vi "VisualizeAppBase.vi"() -> ()   [LabVIEW 2017, in "Visualization.lvlib" / "VisualizeAppBase_class.lvclass"]
uses:
  VisualizeAppBase_class.lvclass
  Modules/AppModule/PublicAPI/Arguments/Broadcasts/clStatUpdate.ctl
  VisializeBase_class/Requests/clUserEventType.ctl
  <vilib>/event_ctls.llb/usereventprio.ctl
  <vilib>/Utility/error.llb/Error Cluster From Error Code.vi
  <vilib>/ErrorRing/Error Ring.xnode
  <userlib>/NIST/NISTErrorLib/NISTErrorLib.lvlib
  VisializeBase_class/VisualizeBase_class.lvclass
  Modules/AppModule/AppModule.lvlib
panel:
  out "Status Broadcasts":string
  out "Error Array":errorcluster[][](array[cluster])
  in  "QueName":string="VisAppQue"
  in  "btnStop":bool
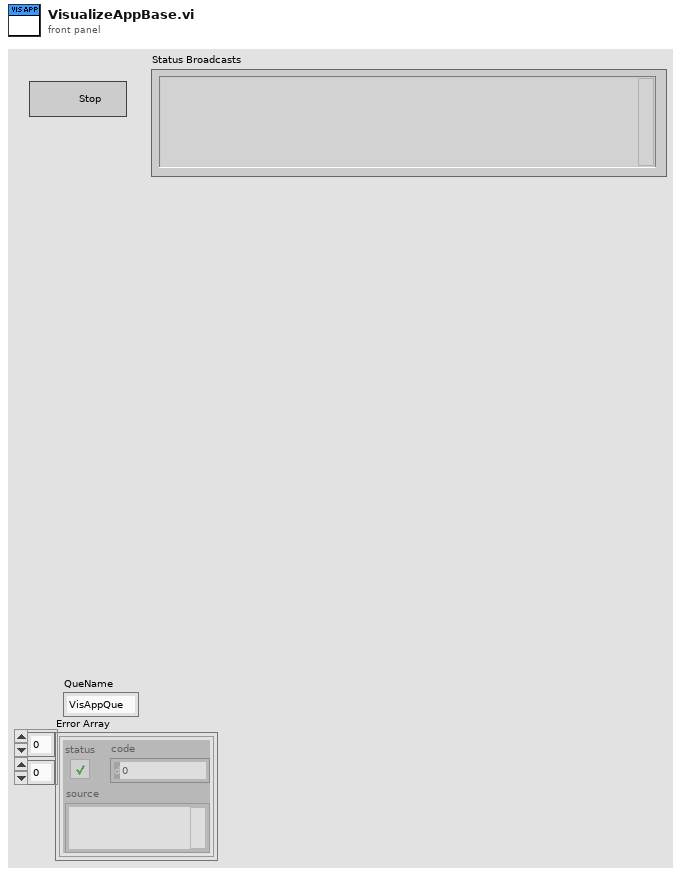
[diagram p1: front panel]
types:
  T1 = typedef "Visualization.lvlib/VisualizeBase_class.lvclass/clRequestEvents.ctl" = cluster{"StopRequest":refnum<user-event>}
  T2 = typedef "AppModule.lvlib/clBroadcastEvents.ctl" = cluster{"DidInit":refnum<user-event>, "StatusUpdate":refnum<user-event>, "ErrorReport":refnum<user-event>, "DidStop":refnum<user-event>, "PathToINI":refnum<user-event>, "InputData":refnum<user-event>, "OutputData":refnum<user-event>, "BcAppInfo":refnum<user-event>, "ConfigData":refnum<user-event>}
  T3 = typedef "Visualization.lvlib/VisualizeBase_class.lvclass/clUserEventType.ctl" = cluster{"BusIndex":i8, "Data":variant}
  T4 = typedef "usereventprio.ctl" = enum32{"high priority", "normal priority"}
  T5 = typedef "AppModule.lvlib/clStatUpdate.ctl" = cluster{"Status":string}
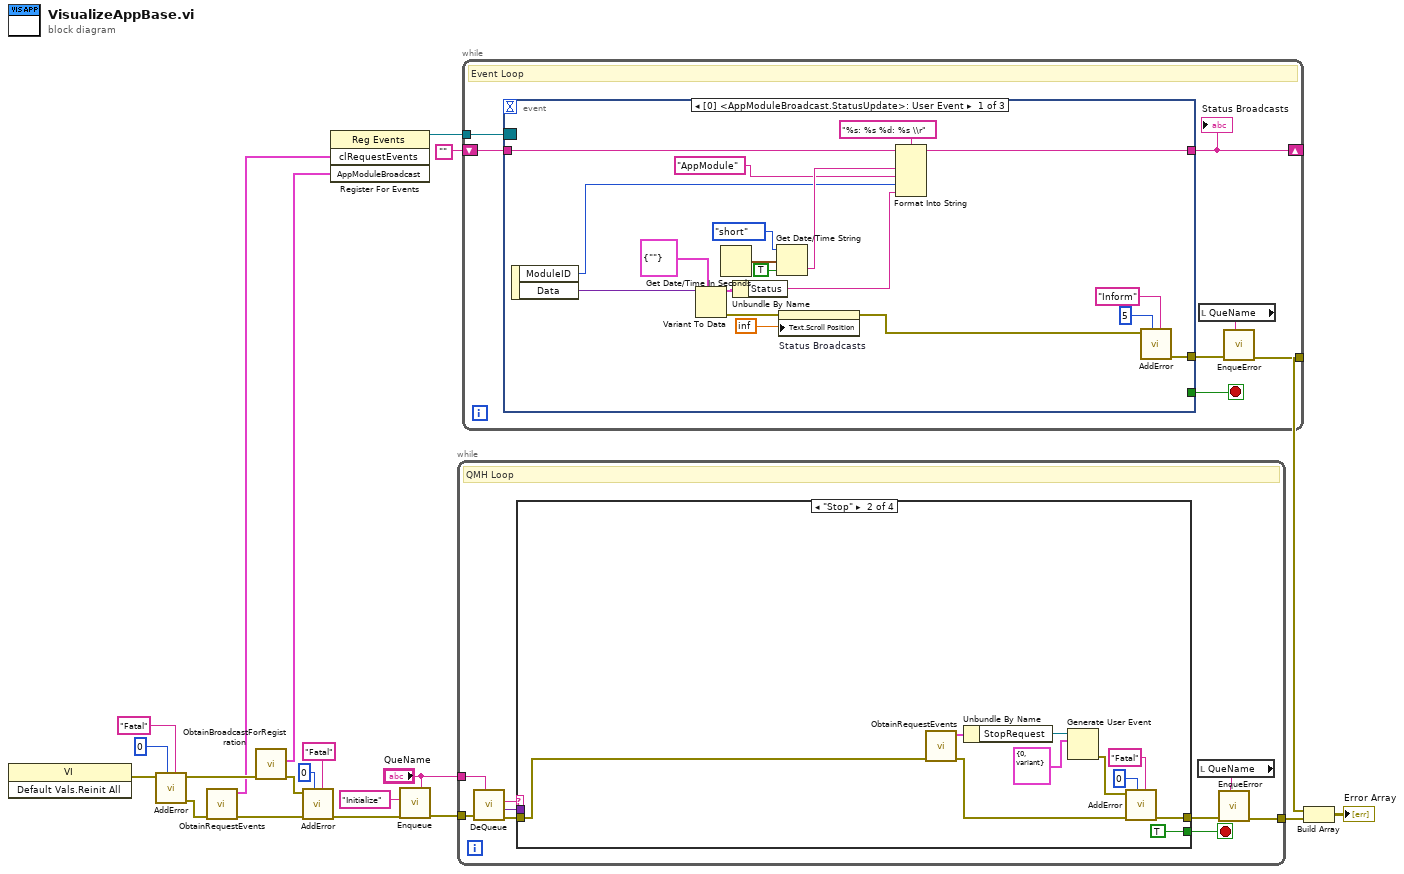
[diagram p0: block diagram]
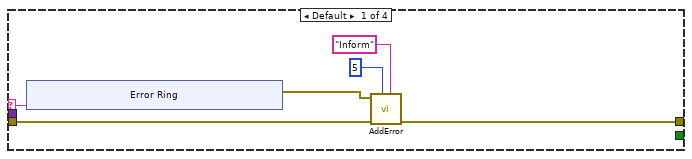
[diagram p2: hidden frame]
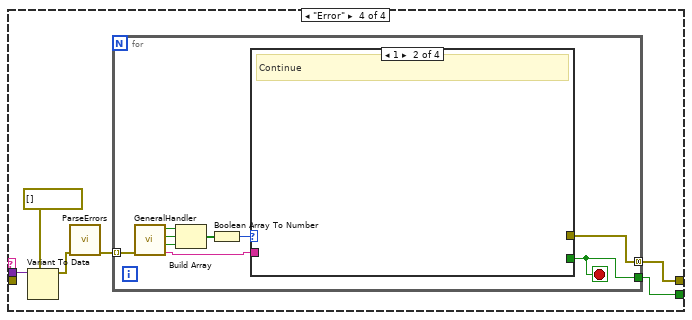
[diagram p4: hidden frame]
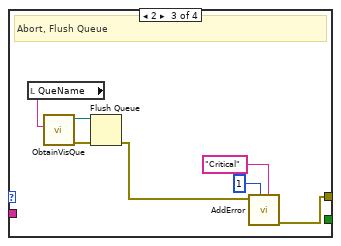
[diagram p6: hidden frame]
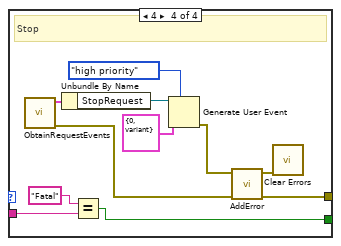
[diagram p7: hidden frame]
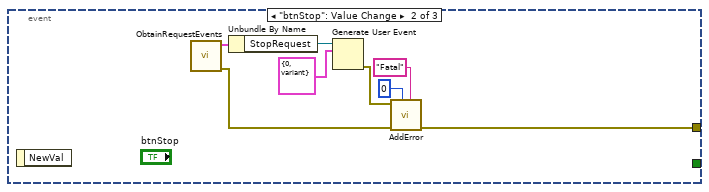
[diagram p8: hidden frame]
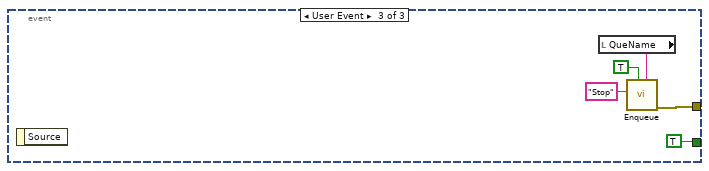
[diagram p9: hidden frame]
diagram:
  n1 = invoke class="VI" method="Default Vals.Reinit All"() -> (error out=w1:errorcluster)  [unwired: 3 in, 2 out]
  n2 = call <userlib>:"AddError.vi"("Severity"="Fatal", "Priority"=u8 0, "error in (no error)"=w1) -> ("ErrorArray"=w18:errorcluster[], "error out"=w17:errorcluster)  [unwired: 7 in]
  n3 = call "ObtainRequestEvents.vi"("Error"=w18) -> ("Error"=w14:errorcluster[], "clRequestEvents"=w16:T1)  [unwired: 9 in]
  n4 = call "ObtainBroadcastForRegistration.vi"("error in (no error)"=w17) -> ("error out"=w11:errorcluster, "AppModuleBroadcast"=w15:T2)  [unwired: 9 in]
  n5 = call <userlib>:"AddError.vi"("Severity"="Fatal", "Priority"=u8 0, "ErrorArray"=w14, "error in (no error)"=w11) -> ("ErrorArray"=w12:errorcluster[])  [unwired: 6 in, 1 out]
  n6 = register-events(w16, w15) -> (reference out=w6:refnum<event-registration>)  [unwired: 2 in, 1 out]
  n7 = call "Enqueue.vi"("QueName"="QueName", "Error"=w12, "Message"="Initialize") -> ("Error"=w8:errorcluster[])  [unwired: 8 in]
  n8 = while {
    tunnel: w8 -> [w29]
    tunnel: "QueName" -> [w28]
    tunnel: [w21] -> w5
    stop <- w24 stop-if-true
    # "QMH Loop"
    n9 = call "DeQueue.vi"("QueName"=w28, "Error"=w29) -> ("Error"=w25:errorcluster[], "Data"=w26:variant, "Message"=w27:string)  [unwired: 7 in]
    n10 = case shown="\"Stop\"" w27 {
      selector: w27 -> [w35 _ _ _]
      tunnel: w26 -> [_ _ _ w56]
      tunnel: w25 -> [w34 w44 w53 _]
      tunnel: [w30 w45 w53 w58] -> w23
      tunnel: [_ TRUE _ w59] -> w24
      frame Default {
        n11 = xnode "Error Ring"("parameter 0"=w35) -> ("error out"=w33:errorcluster)
        n12 = call <userlib>:"AddError.vi"("Severity"="Inform", "Priority"=u8 5, "ErrorArray"=w34, "error in (no error)"=w33) -> ("ErrorArray"=w30:errorcluster[])  [unwired: 6 in, 1 out]
      }
      frame "Stop" {
        n13 = call "ObtainRequestEvents.vi"("Error"=w44) -> ("Error"=w43:errorcluster[], "clRequestEvents"=w46:T1)  [unwired: 9 in]
        n14 = Unbundle By Name(w46) -> ("StopRequest"=w47:refnum<user-event>)
        n15 = Generate User Event(user event=w47, event data cluster=T3 {"BusIndex"=0, "Data"=variant} ("clEventType")) -> (error out=w49:errorcluster)  [unwired: 2 in, 1 out]
        n16 = call <userlib>:"AddError.vi"("Severity"="Fatal", "Priority"=u8 0, "ErrorArray"=w43, "error in (no error)"=w49) -> ("ErrorArray"=w45:errorcluster[])  [unwired: 6 in, 1 out]
      }
      frame "Initialize" {
      }
      frame "Error" {
        n17 = Variant To Data(type=errorcluster[] [], Variant=w56) -> (data=w54:errorcluster[])  [unwired: 1 in, 1 out]
        n18 = call <userlib>:"ParseErrors.vi"("ErrorArray"=w54) -> ("ErrorArray"=w57:errorcluster[])  [unwired: 8 in, 2 out]
        n19 = for {
          tunnel: w57 -> [w68] mode=indexing
          tunnel: [w62] -> w58 mode=concatenating
          tunnel: [w60] -> w59
          stop <- w60 stop-if-true
          n20 = call <userlib>:"GeneralHandler.vi"("error in (no error)"=w68) -> ("Severity"=w61:string, "Stop"=w65:bool, "Abort"=w66:bool, "Continue"=w67:bool)  [unwired: 7 in]
          n21 = Build Array(w67, w66, w65) -> (w64:bool[])
          n22 = Boolean Array To Number(Boolean array=w64) -> (number=w63:u32)
          n23 = case shown="1" w63 {
            tunnel: [_ _ w73 w84] -> w62
            tunnel: w61 -> [_ _ _ w78]
            tunnel: [_ _ _ w76] -> w60
            frame 0, Default {
              # "No Dialog"
            }
            frame 1 {
              # "Continue"
            }
            frame 2 {
              # "Abort, Flush Queue"
              n24 = local read "QueName"() -> (w69:string)
              n25 = call "ObtainVisQue.vi"("QueName"=w69) -> ("error out"=w75:errorcluster, "queue out"=w74:refnum<queue>)  [unwired: 9 in]
              n26 = Flush Queue(queue=w74, error in (no error)=w75) -> (error out=w72:errorcluster)  [unwired: 2 out]
              n27 = call <userlib>:"AddError.vi"("Severity"="Critical" ("String"), "Priority"=u8 1, "error in (no error)"=w72) -> ("ErrorArray"=w73:errorcluster[])  [unwired: 7 in, 1 out]
            }
            frame 4 {
              # "Stop"
              n28 = call "ObtainRequestEvents.vi"() -> ("Error"=w82:errorcluster[], "clRequestEvents"=w86:T1)  [unwired: 10 in]
              n29 = Unbundle By Name(w86) -> ("StopRequest"=w85:refnum<user-event>)
              n30 = Equal?(x="Fatal", y=w78) -> (x = y?=w76:bool)
              n31 = Generate User Event(priority (normal)=usereventprio."high priority", user event=w85, event data cluster=T3 {"BusIndex"=0, "Data"=variant} ("event data")) -> (error out=w83:errorcluster)  [unwired: 1 in, 1 out]
              n32 = call <userlib>:"AddError.vi"("ErrorArray"=w82, "error in (no error)"=w83) -> ("ErrorArray"=w84:errorcluster[], "error out"=w79:errorcluster)  [unwired: 8 in]
              n33 = call <vilib>:"Clear Errors.vi"("error in (no error)"=w79) -> ()  [unwired: 5 in, 2 out]
            }
          }
        }
      }
    }
    n34 = local read "QueName"() -> (w22:string)
    n35 = call "EnqueError.vi"("QueName"=w22, "Error"=w23) -> ("Error"=w21:errorcluster[])  [unwired: 9 in]
  }
  n36 = while {
    tunnel: [w92] -> w4
    tunnel: w6 -> [w90]
    shift-right: [w87] -> _
    shift-left: "" -> [w88]
    stop <- w89 stop-if-true
    # "Event Loop"
    n37 = event shown="[0] <AppModuleBroadcast.StatusUpdate>: User Event" {
      selector: w90 -> [_ _ _]
      dyn-events: _ -> [_ _ _]
      timeout: _ -> [_ _ _]
      tunnel: [w101 w115 w122] -> w93
      tunnel: [_ _ TRUE] -> w89
      tunnel: w88 -> [w112 _ _]
      tunnel: [w105 _ _] -> w87
      event User Event {
        n38 = event-data() -> ("ModuleID"=w95:i32, "Data"=w111:variant)  [unwired: 1 in]
        n39 = Variant To Data(type=T5 {"Status"=""} ("clStatUpdate"), Variant=w111) -> (data=w109:T5, error out=w102:errorcluster)  [unwired: 1 in]
        n40 = Get Date/Time In Seconds() -> (seconds since 1Jan1904=w106:timestamp)
        n41 = Unbundle By Name(w109) -> ("Status"=w96:string)
        n42 = Get Date/Time String(date format (0)=enum16{"short", "long", "abbreviated"}."short", seconds (now)=w106, want seconds? (F)=TRUE) -> (time string=w103:string)  [unwired: 1 out]
        n43 = property on="Status Broadcasts" class="Str"(error in=w102, "Text.Scroll Position"=inf) -> (error out=w100:errorcluster)  [unwired: 1 in, 1 out]
        n44 = Format Into String(format string="%s: %s %d: %s \\r", initial string=w112, w103, "AppModule", w95, w96) -> (resulting string=w105:string)  [unwired: 1 in, 1 out]
        n45 = call <userlib>:"AddError.vi"("Severity"="Inform", "Priority"=u8 5, "error in (no error)"=w100) -> ("ErrorArray"=w101:errorcluster[])  [unwired: 7 in, 1 out]
      }
      event "btnStop": Value Change {
        n46 = event-data() -> ()  [unwired: 1 in, 1 out]
        n47 = call "ObtainRequestEvents.vi"() -> ("Error"=w117:errorcluster[], "clRequestEvents"=w120:T1)  [unwired: 10 in]
        n48 = Unbundle By Name(w120) -> ("StopRequest"=w119:refnum<user-event>)
        n49 = Generate User Event(user event=w119, event data cluster=T3 {"BusIndex"=0, "Data"=variant} ("clEventType")) -> (error out=w116:errorcluster)  [unwired: 2 in, 1 out]
        n50 = call <userlib>:"AddError.vi"("Severity"="Fatal", "Priority"=u8 0, "ErrorArray"=w117, "error in (no error)"=w116) -> ("ErrorArray"=w115:errorcluster[])  [unwired: 6 in, 1 out]
      }
      event User Event {
        n51 = event-data() -> ()  [unwired: 1 in, 1 out]
        n52 = local read "QueName"() -> (w124:string)
        n53 = call "Enqueue.vi"("QueName"=w124, "Priority? (F)"=TRUE, "Message"="Stop") -> ("Error"=w122:errorcluster[])  [unwired: 8 in]
      }
    }
    "Status Broadcasts" <- w87
    n54 = local read "QueName"() -> (w91:string)
    n55 = call "EnqueError.vi"("QueName"=w91, "Error"=w93) -> ("Error"=w92:errorcluster[])  [unwired: 9 in]
  }
  n56 = Build Array(w4, w5) -> (→"Error Array":errorcluster[][])
